vi "TestSequenceSubVI.vi"(0 "GuiRef":T1, 11 "errorin":errorcluster) -> (15 "errorout":errorcluster)   [LabVIEW 2013]
uses:
  Ctl/Paractl.ctl
  GlobValue.vi
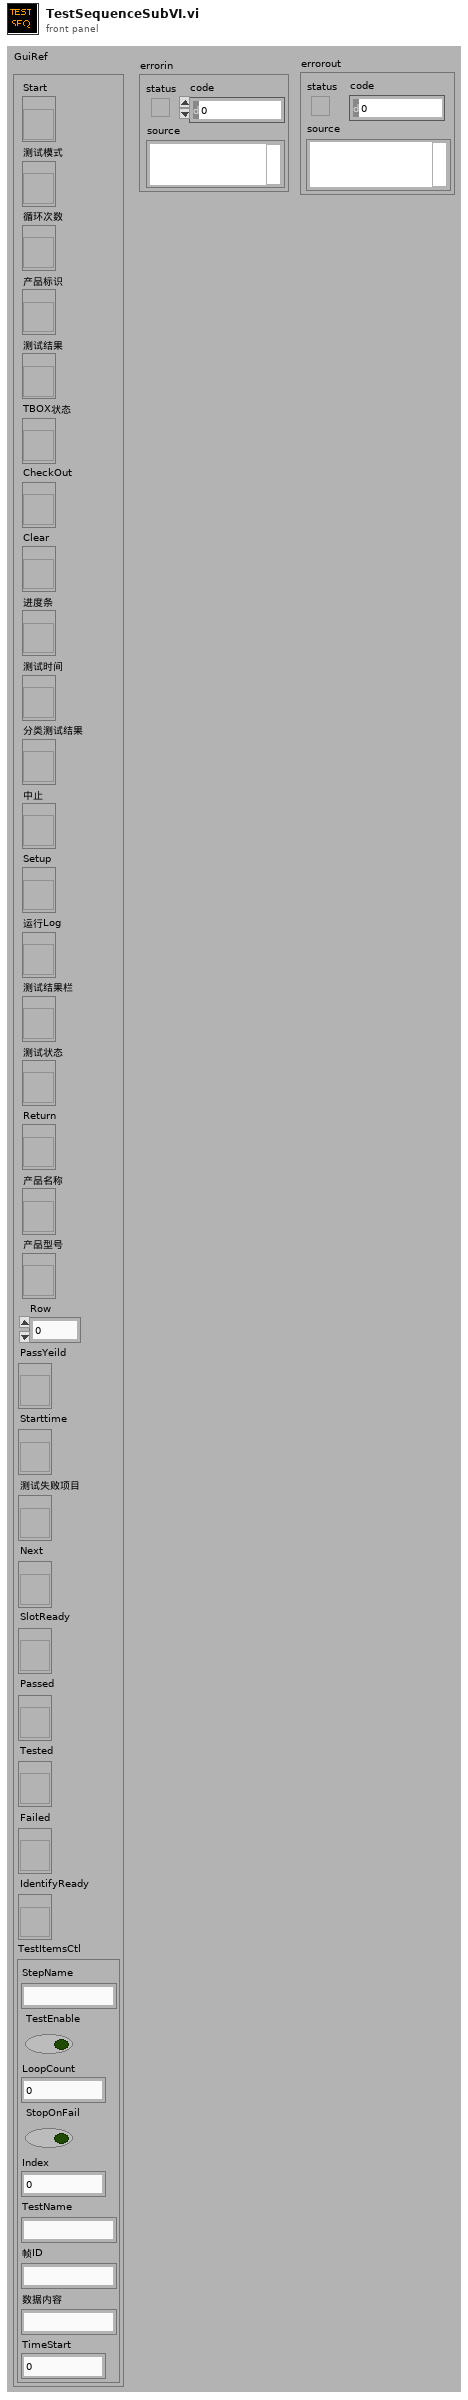
[diagram p1: front panel]
types:
  T1 = typedef "控件.ctl" = cluster{"Start":refnum<vi>, "测试模式":refnum<vi>, "循环次数":refnum<vi>, "产品标识":refnum<vi>, "测试结果":refnum<vi>, "TBOX状态":refnum<vi>, "CheckOut":refnum<vi>, "Clear":refnum<vi>, "进度条":refnum<vi>, "测试时间":refnum<vi>, "分类测试结果":refnum<vi>, "中止":refnum<vi>, "Setup":refnum<vi>, "运行Log":refnum<vi>, "测试结果栏":refnum<vi>, "测试状态":refnum<vi>, "Return":refnum<vi>, "产品名称":refnum<vi>, "产品型号":refnum<vi>, "Row":i32, "PassYeild":refnum<vi>, "Starttime":refnum<vi>, "测试失败项目":refnum<vi>, "Next":refnum<vi>, "SlotReady":refnum<vi>, "Passed":refnum<vi>, "Tested":refnum<vi>, "Failed":refnum<vi>, "IdentifyReady":refnum<vi>, "TestItemsCtl":cluster{"StepName":string, "TestEnable":bool, "LoopCount":u32, "StopOnFail":bool, "Index":u32, "TestName":string, "帧ID":string, "数据内容":string, "TimeStart":u32}}
  T2 = typedef "Paractl.ctl" = enum16{"Fw Ver", "HW Ver", "CCID", "WiFiName", "DevID", "SN", "TUID", "CertifID", "PdTime", "Provider", "WiFiPassword", "Imei", "AuthCode", "Reserved1", "Reserved2", "Reserved3"}
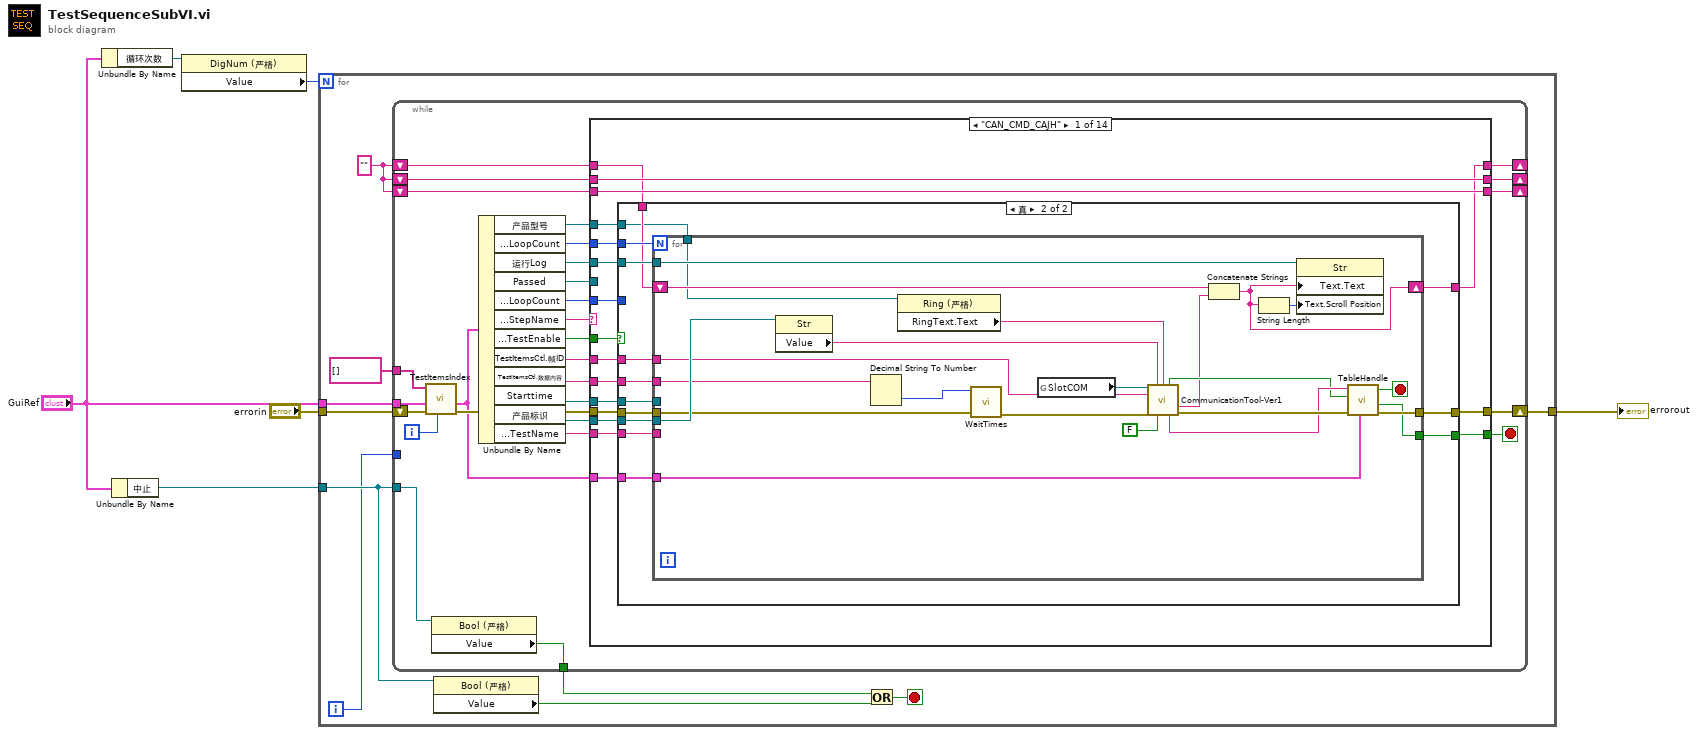
[diagram p0: block diagram]
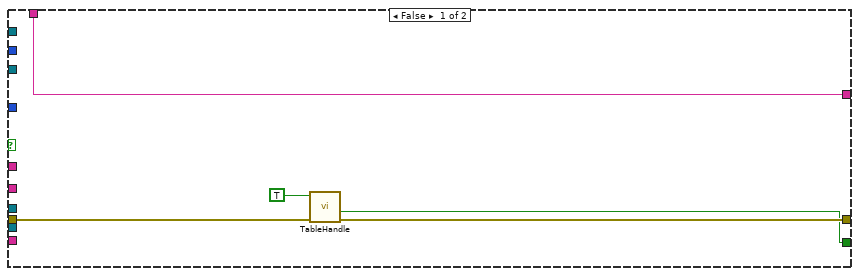
[diagram p2: hidden frame]
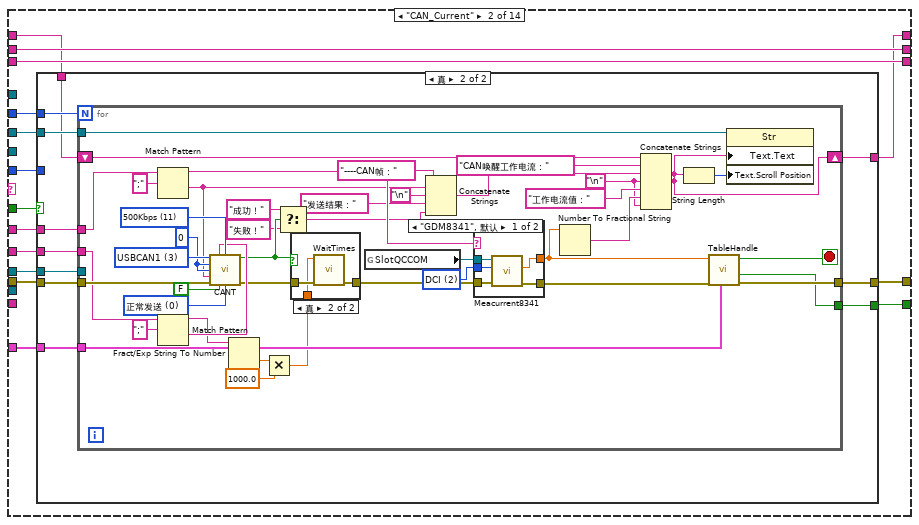
[diagram p3: hidden frame]
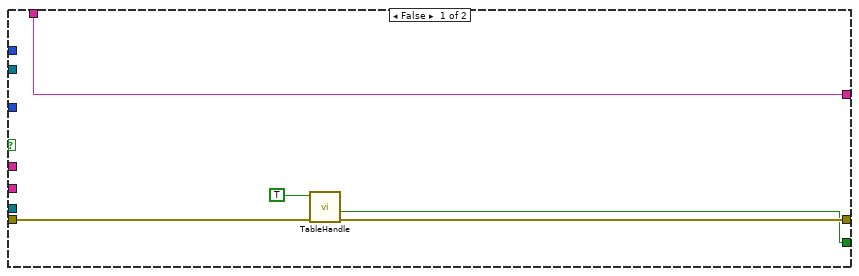
[diagram p4: hidden frame]
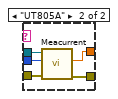
[diagram p6: hidden frame]
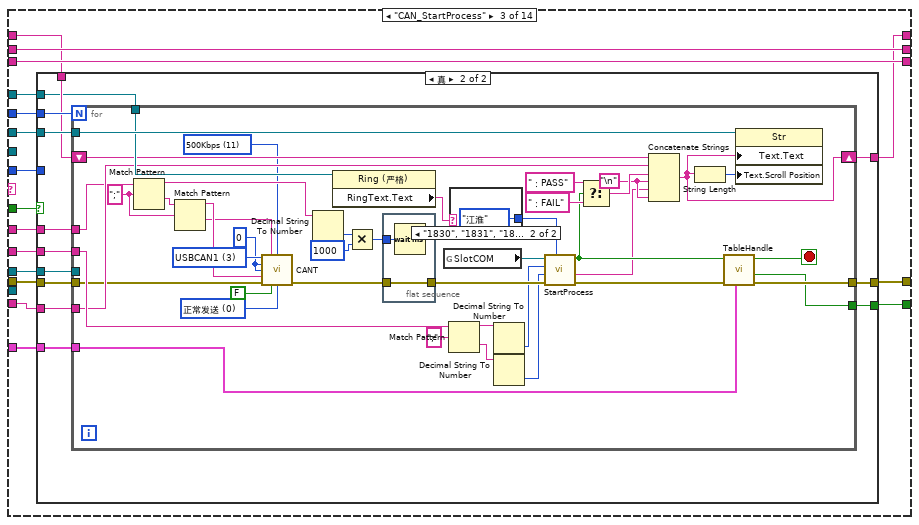
[diagram p7: hidden frame]
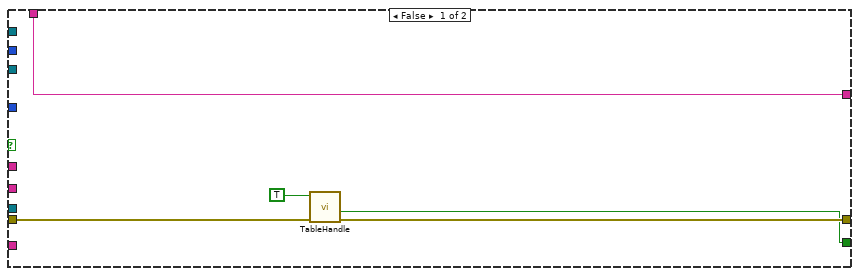
[diagram p8: hidden frame]
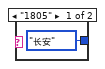
[diagram p9: hidden frame]
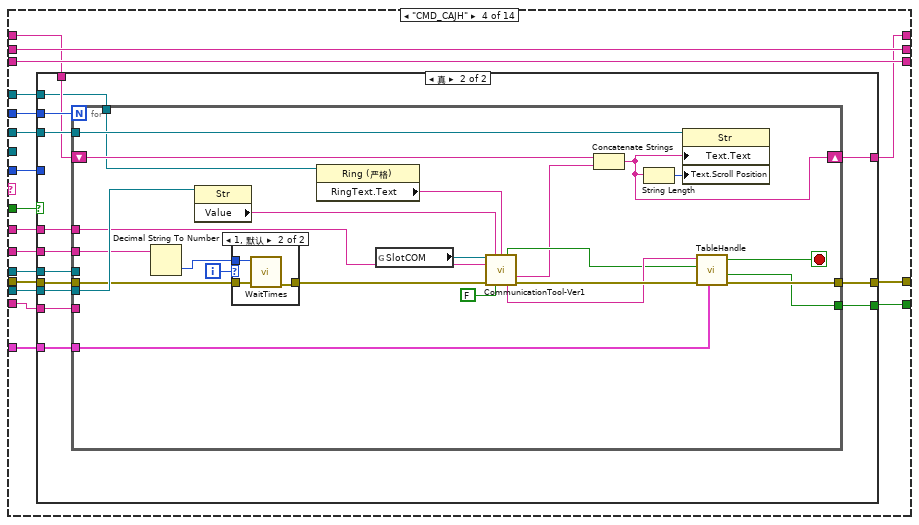
[diagram p10: hidden frame]
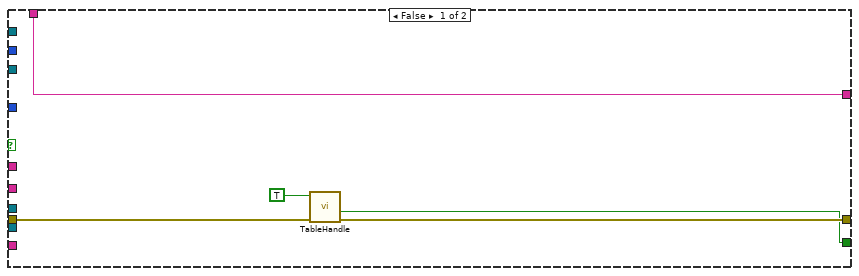
[diagram p11: hidden frame]
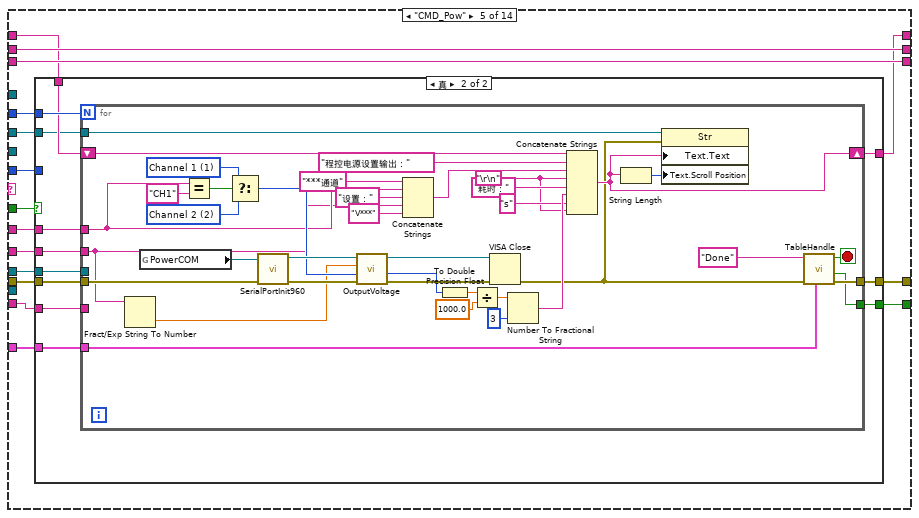
[diagram p13: hidden frame]
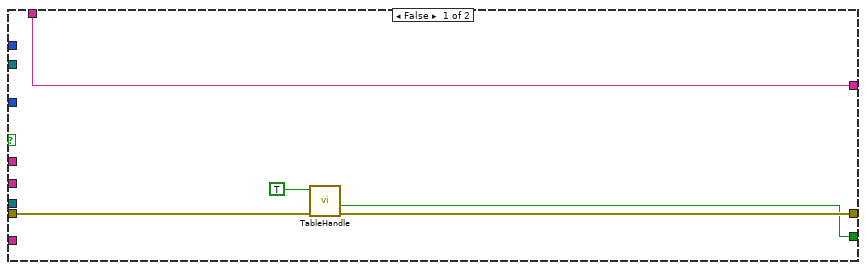
[diagram p14: hidden frame]
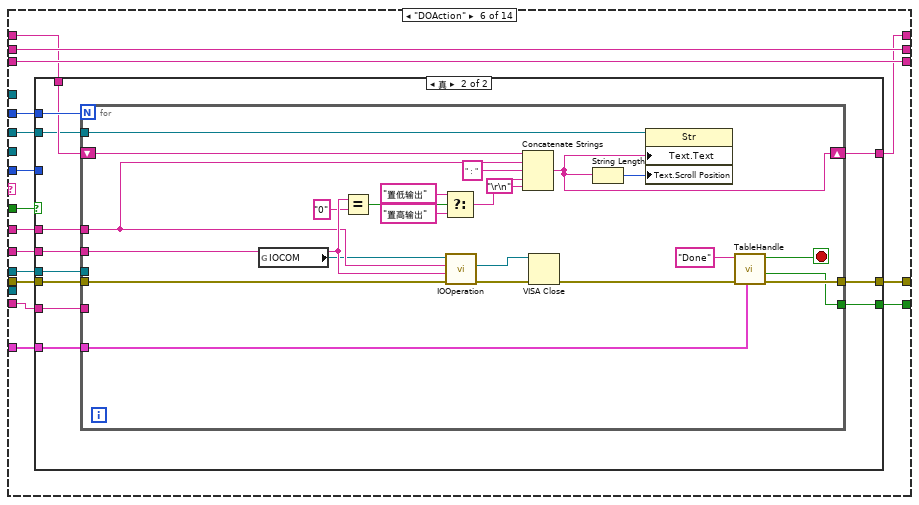
[diagram p15: hidden frame]
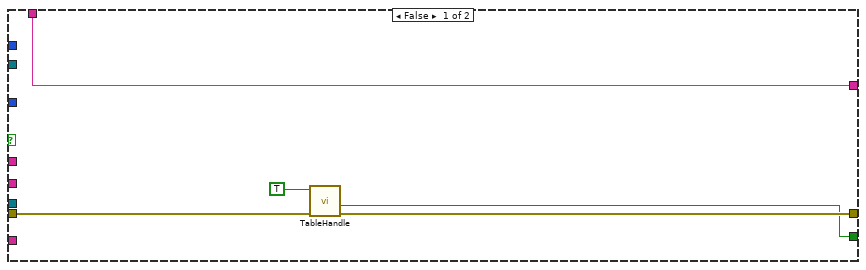
[diagram p16: hidden frame]
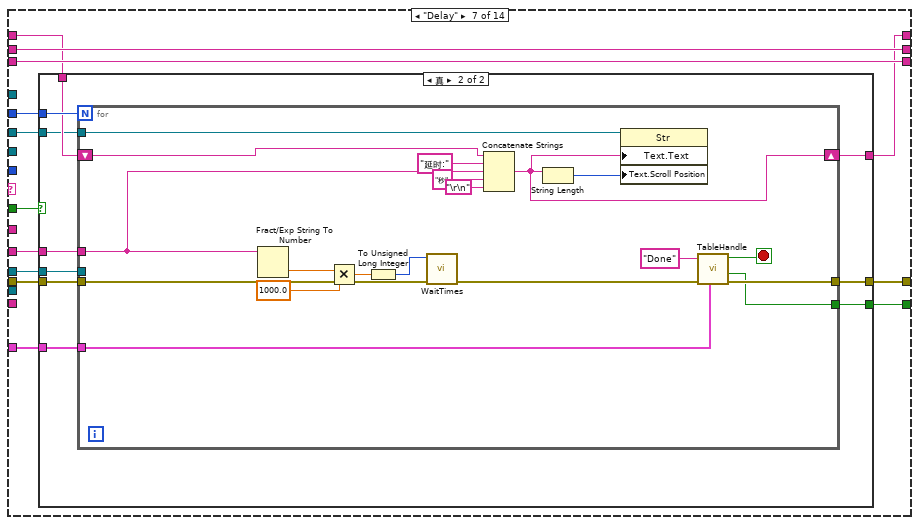
[diagram p17: hidden frame]
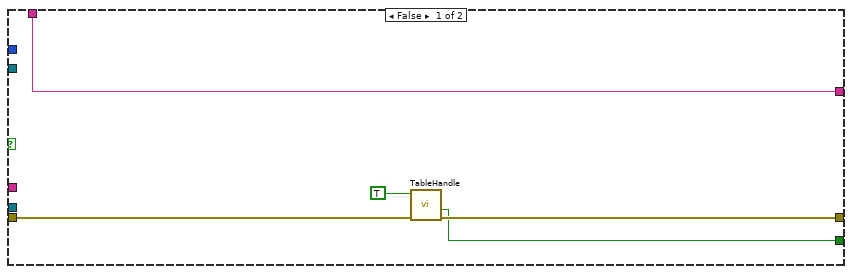
[diagram p18: hidden frame]
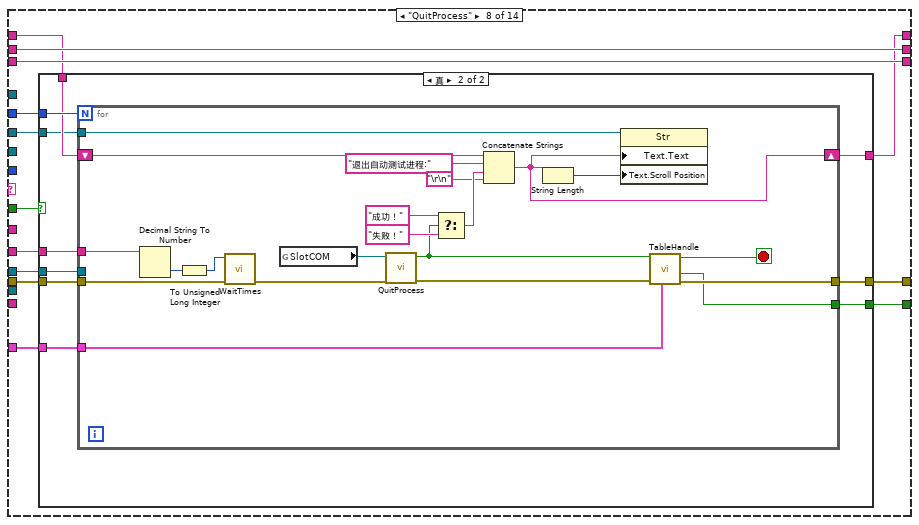
[diagram p19: hidden frame]
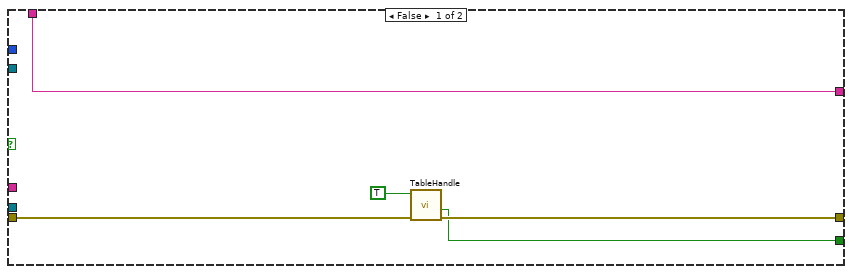
[diagram p20: hidden frame]
diagram:
  n1 = Unbundle By Name("GuiRef") -> ("循环次数"=w4:refnum<vi>)
  n2 = Unbundle By Name("GuiRef") -> ("中止"=w1:refnum<vi>)
  n3 = property class="DigNum (严格)"(reference=w4) -> ("Value"=w3:u32)  [unwired: 1 in, 2 out]
  n4 = for {
    N: w3 -> [_]
    tunnel: [w16] -> w6
    tunnel: "errorin" -> [w15]
    tunnel: "GuiRef" -> [w14]
    tunnel: w1 -> [w11]
    i -> [w7]
    stop <- w8 stop-if-true
    w12 = "" ("CMD")
    n5 = while {
      shift-right: [w40] -> w16
      shift-left: w15 -> [w44]
      tunnel: w14 -> [w19]
      shift-right: [w31] -> _
      shift-left: w12 -> [w30]
      tunnel: string[] [] ("Fail项目") -> [w29]
      shift-right: [w27] -> _
      shift-left: w12 -> [w26]
      shift-right: [w24] -> _
      shift-left: w12 -> [w25]
      tunnel: w11 -> [w18]
      tunnel: [w17] -> w10
      tunnel: w7 -> [_]
      i -> [w28]
      stop <- w39 stop-if-true
      n6 = call "TestItemsIndex.vi"("TestItemIndexIn"=w28, "ErrorIn"=w44, "GuiRef"=w19, "Fail项目"=w29) -> ("ErrorOut"=w43:errorcluster, "GuiRefOut"=w38:T1)  [unwired: 6 in]
      n7 = property class="Bool (严格)"(reference=w18) -> ("Value"=w17:bool)  [unwired: 1 in, 2 out]
      n8 = Unbundle By Name(w38) -> ("产品型号"=w21:refnum<vi>, "TestItemsCtl.LoopCount"=w23:u32, "运行Log"=w32:refnum<vi>, "Passed"=w33:refnum<vi>, "TestItemsCtl.LoopCount"=w34:u32, "TestItemsCtl.StepName"=w42:string, "TestItemsCtl.TestEnable"=w41:bool, "TestItemsCtl.帧ID"=w35:string, "TestItemsCtl.数据内容"=w36:string, "Starttime"=w37:refnum<vi>, "产品标识"=w22:refnum<vi>, "TestItemsCtl.TestName"=w20:string)
      n9 = case shown="\"CAN_CMD_CAJH\"" w42 {
        selector: w42 -> [_ _ _ _ _ _ _ _ _ _ _ _ _ w788]
        tunnel: [w53 w110 w200 w283 w353 w424 w477 w524 w570 w643 w700 w713 w780 w790] -> w40
        tunnel: w43 -> [w57 w114 w204 w287 w354 w425 w478 w525 w574 w647 w700 w714 w780 _]
        tunnel: w38 -> [w56 w113 w203 w286 w355 w426 w479 w526 w573 w646 _ w715 _ _]
        tunnel: w41 -> [w52 w109 w199 w282 w352 w423 w476 w523 w569 w642 _ w712 _ _]
        tunnel: [w54 w111 w201 w284 w351 w422 w475 w522 w571 w644 TRUE ("StopOnFail?") w711 FALSE ("StopOnFail?") TRUE ("StopOnFail?")] -> w39
        tunnel: w37 -> [w55 w112 w202 w285 w350 w421 w474 w521 w572 w645 _ w710 _ _]
        tunnel: w36 -> [w58 w115 w205 w288 w348 w419 w473 w520 w575 w648 _ w708 _ _]
        tunnel: w35 -> [w59 w116 w206 w289 w349 w420 _ _ w576 w649 _ w709 _ _]
        tunnel: w34 -> [w60 w117 w207 w290 w347 w418 _ _ w577 w650 _ _ _ _]
        tunnel: w33 -> [_ _ _ _ _ _ _ _ _ _ _ _ _ _]
        tunnel: w32 -> [w51 w108 w198 w281 w342 w413 w468 w515 w568 w641 _ w704 _ _]
        tunnel: [w48 w105 w195 w278 w340 w411 w467 w514 w565 w638 w698 w703 w778 w785] -> w31
        tunnel: w30 -> [w49 w106 w196 w279 w343 w414 w469 w516 w566 w639 w698 w705 w778 w785]
        tunnel: [w62 w119 w209 w292 w346 w417 w472 w519 w579 w652 w697 w707 w777 w782] -> w27
        tunnel: w26 -> [w62 w119 w209 w292 w346 w417 w472 w519 w579 w652 w697 w707 w777 w782]
        tunnel: w25 -> [w61 w118 w208 w291 w345 w416 w471 w518 w578 w651 w696 w706 w776 w781]
        tunnel: [w61 w118 w208 w291 w345 w416 w471 w518 w578 w651 w696 w706 w776 w781] -> w24
        tunnel: w23 -> [w50 w107 w197 w280 w344 w415 w470 w517 w567 w640 _ w701 _ _]
        tunnel: w22 -> [w45 _ _ w275 _ _ _ _ _ _ _ _ _ _]
        tunnel: w21 -> [w47 _ w194 w277 _ _ _ _ w564 _ _ w702 _ _]
        tunnel: w20 -> [w46 _ w193 w276 w341 w412 _ _ w563 _ _ _ _ _]
        frame "CAN_CMD_CAJH" {
          n10 = case shown="真" w52 {
            tunnel: w56 -> [_ w79]
            tunnel: w57 -> [w66 w81]
            tunnel: [w67 w80] -> w53
            tunnel: [w65 w78] -> w54
            tunnel: w55 -> [_ w77]
            tunnel: w59 -> [_ w76]
            tunnel: w58 -> [_ w75]
            tunnel: w60 -> [_ _]
            tunnel: w51 -> [_ w74]
            tunnel: w50 -> [_ w73]
            tunnel: w49 -> [w63 w72]
            tunnel: [w63 w71] -> w48
            tunnel: w47 -> [_ w70]
            tunnel: w46 -> [_ w69]
            tunnel: w45 -> [_ w68]
            frame False {
              n11 = call "TableHandle.vi"("error in"=w66, "DataIn"=TRUE) -> ("error out"=w67:errorcluster, "Stop?"=w65:bool)  [unwired: 4 in, 4 out]
            }
            frame True {
              n12 = for "For循环" {
                N: w73 -> [_]
                tunnel: w81 -> [w86]
                tunnel: [w104] -> w80
                tunnel: w79 -> [w82]
                tunnel: [w102] -> w78
                tunnel: w77 -> [_]
                tunnel: w75 -> [w84]
                tunnel: w76 -> [w92]
                tunnel: w74 -> [w101]
                shift-right: [w98] -> w71
                shift-left: w72 -> [w100]
                tunnel: w70 -> [w96]
                tunnel: w69 -> [_]
                tunnel: w68 -> [w94]
                stop <- w103 stop-if-true
                n13 = property class="Str"(reference=w94) -> ("Value"=w93:string)  [unwired: 1 in, 2 out]
                n14 = Decimal String To Number(string=w84) -> (number=w83:i32)  [unwired: 2 in, 1 out]
                n15 = property class="Ring (严格)"(reference=w96) -> ("RingText.Text"=w95:string)  [unwired: 1 in, 2 out]
                n16 = call "WaitTimes.vi"("error in (no error)"=w86, "WaitTimes"=w83) -> ("error out"=w85:errorcluster)  [unwired: 9 in]
                n17 = global read "GlobValue.vi" "SlotCOM"() -> (w91:refnum<visa-resource-name>)
                n18 = call "CommunicationTool-Ver1.vi"("VISA资源名称"=w91, "SN"=w93, "ModelNumber"=w95, "通信协议名称"=w92, "error in"=w85, "Debug"=FALSE) -> ("字符串数值"=w88:bool, "CMD"=w87:string, "data"=w89:string, "error out"=w97:errorcluster)  [unwired: 4 in, 2 out]
                n19 = Concatenate Strings(w100, w87) -> (w98:string)
                n20 = String Length(string=w98) -> (length=w99:i32)
                n21 = property class="Str"(reference=w101, "Text.Text"=w98, "Text.Scroll Position"=w99) -> ()  [unwired: 1 in, 2 out]
                n22 = call "TableHandle.vi"("All"=w82, "error in"=w97, "字符串数值"=w88, "DataIn"=w89) -> ("error out"=w104:errorcluster, "Stop?"=w102:bool, "StopForLoop"=w103:bool)  [unwired: 3 in, 2 out]
              }
            }
          }
        }
        frame "CAN_Current" {
          n23 = case shown="真" w109 {
            tunnel: w113 -> [_ w133]
            tunnel: w114 -> [w123 w135]
            tunnel: [w124 w134] -> w110
            tunnel: [w122 w132] -> w111
            tunnel: w112 -> [_ w131]
            tunnel: w116 -> [_ w130]
            tunnel: w115 -> [_ w129]
            tunnel: w117 -> [_ _]
            tunnel: w108 -> [_ w128]
            tunnel: w107 -> [_ w127]
            tunnel: w106 -> [w120 w126]
            tunnel: [w120 w125] -> w105
            frame False {
              n24 = call "TableHandle.vi"("error in"=w123, "DataIn"=TRUE) -> ("error out"=w124:errorcluster, "Stop?"=w122:bool)  [unwired: 4 in, 4 out]
            }
            frame True {
              n25 = for "For循环" {
                N: w127 -> [_]
                tunnel: w135 -> [w166]
                tunnel: [w178] -> w134
                tunnel: w133 -> [w154]
                tunnel: [w176] -> w132
                tunnel: w131 -> [_]
                tunnel: w129 -> [w157]
                tunnel: w130 -> [w160]
                tunnel: w128 -> [w172]
                shift-right: [w167] -> w125
                shift-left: w126 -> [w171]
                stop <- w177 stop-if-true
                w136 = "\n"
                w158 = u32 11 items=["5Kbps", "10Kbps", "20Kbps", "40Kbps", "50Kbps", "80Kbps", "100Kbps", "125Kbps", "200Kbps", "250Kbps", "400Kbps", "500Kbps", "666Kbps", "800Kbps", "1000Kbps"] ("Baud")
                w162 = u8 0 items=["正常发送", "单次发送", "自发自收", "单次自发自收"] ("发送类型")
                w164 = u32 0 ("DevIndex")
                w165 = u32 3 items=["PCI5121"=1, "PCI9810"=2, "USBCAN1"=3, "USBCAN2"=4, "PCI9820"=5, "PCI5110"=7, "PC104CAN"=11, "CANETUDP"=12, "PCI9840B"=14, "PC104C2"=15, "PCI9820I"=16, "CANETTCP"=17, "PCIE9221"=24, "PCI5010U"=19, "USBCAN_E_U"=20, "USBCAN_2E_U"=21, "PCI5020U"=22] ("设备类型")
                w174 = u16 2 items=["DCV", "ACV", "DCI", "ACI", "OHM", "RST", "CAP", "FRQ", "AUTO"] ("测试类型")
                n26 = Match Pattern(string=w160, regular expression=";" ("正则表达式")) -> (before substring=w159:string, after substring=w146:string)  [unwired: 1 in, 2 out]
                n27 = Match Pattern(string=w157, regular expression=";" ("正则表达式")) -> (before substring=w151:string, after substring=w155:string)  [unwired: 1 in, 2 out]
                n28 = call "CANT.vi"("设备类型"=w165, "数据输入"=w155, "Baud"=w158, "DevIndex"=w164, "CANInd"=w164, "ID"=w146, "error in"=w166, "滤波"=FALSE, "发送类型"=w162) -> ("Result"=w145:bool, "error out"=w153:errorcluster)  [unwired: 4 in, 1 out]
                n29 = Fract/Exp String To Number(string=w151) -> (number=w150:dbl)  [unwired: 3 in, 1 out]
                n30 = Multiply(x=w150, y=1000.0) -> (x*y=w148:dbl)
                n31 = Select(t="成功！" ("正则表达式"), s=w145, f="失败！" ("正则表达式")) -> (s? t:f=w140:string)
                n32 = case shown="真" w145 {
                  tunnel: w153 -> [w179 w182]
                  tunnel: [w179 w181] -> w152
                  tunnel: w148 -> [_ w180]
                  frame False {
                  }
                  frame True {
                    n33 = call "WaitTimes.vi"("error in (no error)"=w182, "WaitTimes"=w180) -> ("error out"=w181:errorcluster)  [unwired: 9 in]
                  }
                }
                n34 = global read "GlobValue.vi" "SlotQCCOM"() -> (w175:refnum<visa-resource-name>)
                n35 = Concatenate Strings("----CAN帧：" ("字符串"), w146, "\n", "发送结果：" ("字符串"), w140) -> (w139:string)
                n36 = case shown="\"GDM8341\", 默认" w159 {
                  tunnel: w175 -> [w183 w188]
                  tunnel: w174 -> [w187 w192]
                  tunnel: [w186 w191] -> w169
                  tunnel: [w185 w190] -> w173
                  tunnel: w152 -> [w184 w189]
                  frame "GDM8341", Default {
                    n37 = call "Meacurrent8341.vi"("error in"=w184, "测试类型"=w187, "VISA资源名称"=w183) -> ("错误输出"=w185:errorcluster, "数值"=w186:dbl)  [unwired: 6 in, 1 out]
                  }
                  frame "UT805A" {
                    n38 = call "Meacurrent.vi"("error in"=w189, "测试类型"=w192, "VISA"=w188) -> ("error out"=w190:errorcluster, "数值"=w191:dbl)  [unwired: 7 in]
                  }
                }
                n39 = Number To Fractional String(number=w169) -> (F-format string=w137:string)  [unwired: 3 in]
                n40 = Concatenate Strings(w171, "CAN唤醒工作电流：" ("字符串"), w139, w136, "工作电流值：" ("字符串"), w137, w136) -> (w167:string)
                n41 = String Length(string=w167) -> (length=w168:i32)
                n42 = call "TableHandle.vi"("All"=w154, "error in"=w173, "DataIn"=w169) -> ("error out"=w178:errorcluster, "Stop?"=w176:bool, "StopForLoop"=w177:bool)  [unwired: 4 in, 2 out]
                n43 = property class="Str"(reference=w172, "Text.Text"=w167, "Text.Scroll Position"=w168) -> ()  [unwired: 1 in, 2 out]
              }
            }
          }
        }
        frame "CAN_StartProcess" {
          n44 = case shown="真" w199 {
            tunnel: w203 -> [_ w225]
            tunnel: w204 -> [w213 w227]
            tunnel: [w214 w226] -> w200
            tunnel: [w212 w224] -> w201
            tunnel: w202 -> [_ w223]
            tunnel: w206 -> [_ w222]
            tunnel: w205 -> [_ w221]
            tunnel: w207 -> [_ _]
            tunnel: w198 -> [_ w220]
            tunnel: w197 -> [_ w219]
            tunnel: w196 -> [w210 w218]
            tunnel: [w210 w217] -> w195
            tunnel: w194 -> [_ w216]
            tunnel: w193 -> [_ w215]
            frame False {
              n45 = call "TableHandle.vi"("error in"=w213, "DataIn"=TRUE) -> ("error out"=w214:errorcluster, "Stop?"=w212:bool)  [unwired: 4 in, 4 out]
            }
            frame True {
              n46 = for "For循环" {
                N: w219 -> [_]
                tunnel: w227 -> [w239]
                tunnel: [w270] -> w226
                tunnel: w225 -> [w228]
                tunnel: [w268] -> w224
                tunnel: w223 -> [_]
                tunnel: w221 -> [w257]
                tunnel: w222 -> [w243]
                tunnel: w220 -> [w267]
                shift-right: [w245] -> w217
                shift-left: w218 -> [w249]
                tunnel: w216 -> [w263]
                tunnel: w215 -> [w248]
                stop <- w269 stop-if-true
                w232 = u32 11 items=["5Kbps", "10Kbps", "20Kbps", "40Kbps", "50Kbps", "80Kbps", "100Kbps", "125Kbps", "200Kbps", "250Kbps", "400Kbps", "500Kbps", "666Kbps", "800Kbps", "1000Kbps"] ("Baud")
                w237 = u8 0 items=["正常发送", "单次发送", "自发自收", "单次自发自收"] ("发送类型")
                w240 = u32 0 ("DevIndex")
                w241 = u32 3 items=["PCI5121"=1, "PCI9810"=2, "USBCAN1"=3, "USBCAN2"=4, "PCI9820"=5, "PCI5110"=7, "PC104CAN"=11, "CANETUDP"=12, "PCI9840B"=14, "PC104C2"=15, "PCI9820I"=16, "CANETTCP"=17, "PCIE9221"=24, "PCI5010U"=19, "USBCAN_E_U"=20, "USBCAN_2E_U"=21, "PCI5020U"=22] ("设备类型")
                w235 = ";"
                w251 = "\n"
                n47 = Match Pattern(string=w243, regular expression=w235) -> (before substring=w242:string, after substring=w236:string)  [unwired: 1 in, 2 out]
                n48 = Match Pattern(string=w236, regular expression=w235) -> (before substring=w234:string, after substring=w233:string)  [unwired: 1 in, 2 out]
                n49 = call "CANT.vi"("设备类型"=w241, "数据输入"=w233, "Baud"=w232, "DevIndex"=w240, "CANInd"=w240, "ID"=w234, "error in"=w239, "滤波"=FALSE, "发送类型"=w237) -> ("error out"=w244:errorcluster)  [unwired: 4 in, 2 out]
                n50 = Decimal String To Number(string=w242) -> (number=w231:i32)  [unwired: 2 in, 1 out]
                n51 = property class="Ring (严格)"(reference=w263) -> ("RingText.Text"=w264:string)  [unwired: 1 in, 2 out]
                n52 = Multiply(x=w231, y=1000) -> (x*y=w229:i32)
                n53 = flat-sequence {
                  tunnel: [w272] -> w261
                  tunnel: w244 -> [w272]
                  tunnel: w229 -> [w271]
                  frame #0 {
                    n54 = Wait (ms)(milliseconds to wait=w271) -> ()  [unwired: 1 out]
                  }
                }
                n55 = global read "GlobValue.vi" "SlotCOM"() -> (w265:refnum<visa-resource-name>)
                n56 = Match Pattern(string=w257, regular expression=";") -> (before substring=w259:string, after substring=w258:string)  [unwired: 1 in, 2 out]
                n57 = case shown="\"1830\", \"1831\", \"1832\", 默认" w264 {
                  tunnel: [enum16{"长安", "江淮"}."长安" ("型号") enum16{"长安", "江淮"}."江淮" ("型号")] -> w262
                  frame "1805" {
                  }
                  frame "1830", "1831", "1832", Default {
                  }
                }
                n58 = Decimal String To Number(string=w259) -> (number=w256:i32)  [unwired: 2 in, 1 out]
                n59 = Decimal String To Number(string=w258) -> (number=w255:i32)  [unwired: 2 in, 1 out]
                n60 = call "StartProcess.vi"("型号"=w262, "error in"=w261, "延时"=w255, "Cycles"=w256, "COMIn"=w265) -> ("error out"=w266:errorcluster, "连接的字符串"=w247:string, "OK？"=w250:bool)  [unwired: 3 in, 1 out]
                n61 = Select(t="：PASS", s=w250, f="：FAIL") -> (s? t:f=w252:string)
                n62 = Concatenate Strings(w249, w248, w252, w251, w247, w251) -> (w245:string)
                n63 = String Length(string=w245) -> (length=w246:i32)
                n64 = call "TableHandle.vi"("All"=w228, "error in"=w266, "DataIn"=w250) -> ("error out"=w270:errorcluster, "Stop?"=w268:bool, "StopForLoop"=w269:bool)  [unwired: 4 in, 2 out]
                n65 = property class="Str"(reference=w267, "Text.Text"=w245, "Text.Scroll Position"=w246) -> ()  [unwired: 1 in, 2 out]
              }
            }
          }
        }
        frame "CMD_CAJH" {
          n66 = case shown="真" w282 {
            tunnel: w286 -> [_ w309]
            tunnel: w287 -> [w296 w311]
            tunnel: [w297 w310] -> w283
            tunnel: [w295 w308] -> w284
            tunnel: w285 -> [_ w307]
            tunnel: w289 -> [_ w306]
            tunnel: w288 -> [_ w305]
            tunnel: w290 -> [_ _]
            tunnel: w281 -> [_ w304]
            tunnel: w280 -> [_ w303]
            tunnel: w279 -> [w293 w302]
            tunnel: [w293 w301] -> w278
            tunnel: w277 -> [_ w300]
            tunnel: w276 -> [_ w299]
            tunnel: w275 -> [_ w298]
            frame False {
              n67 = call "TableHandle.vi"("error in"=w296, "DataIn"=TRUE) -> ("error out"=w297:errorcluster, "Stop?"=w295:bool)  [unwired: 4 in, 4 out]
            }
            frame True {
              n68 = for "For循环" {
                N: w303 -> [_]
                tunnel: w311 -> [w317]
                tunnel: [w335] -> w310
                tunnel: w309 -> [w312]
                tunnel: [w333] -> w308
                tunnel: w307 -> [_]
                tunnel: w305 -> [w314]
                tunnel: w306 -> [w323]
                tunnel: w304 -> [w332]
                shift-right: [w329] -> w301
                shift-left: w302 -> [w331]
                tunnel: w300 -> [w327]
                tunnel: w299 -> [_]
                tunnel: w298 -> [w325]
                i -> [w315]
                stop <- w334 stop-if-true
                n69 = Decimal String To Number(string=w314) -> (number=w313:i32)  [unwired: 2 in, 1 out]
                n70 = property class="Str"(reference=w325) -> ("Value"=w324:string)  [unwired: 1 in, 2 out]
                n71 = case shown="1, 默认" w315 {
                  tunnel: w317 -> [w336 w339]
                  tunnel: [w336 w338] -> w316
                  tunnel: w313 -> [_ w337]
                  frame 0 {
                  }
                  frame 1, Default {
                    n72 = call "WaitTimes.vi"("error in (no error)"=w339, "WaitTimes"=w337) -> ("error out"=w338:errorcluster)  [unwired: 9 in]
                  }
                }
                n73 = property class="Ring (严格)"(reference=w327) -> ("RingText.Text"=w326:string)  [unwired: 1 in, 2 out]
                n74 = global read "GlobValue.vi" "SlotCOM"() -> (w322:refnum<visa-resource-name>)
                n75 = call "CommunicationTool-Ver1.vi"("VISA资源名称"=w322, "SN"=w324, "ModelNumber"=w326, "通信协议名称"=w323, "error in"=w316, "Debug"=FALSE) -> ("字符串数值"=w319:bool, "CMD"=w318:string, "data"=w320:string, "error out"=w328:errorcluster)  [unwired: 4 in, 2 out]
                n76 = Concatenate Strings(w331, w318) -> (w329:string)
                n77 = String Length(string=w329) -> (length=w330:i32)
                n78 = property class="Str"(reference=w332, "Text.Text"=w329, "Text.Scroll Position"=w330) -> ()  [unwired: 1 in, 2 out]
                n79 = call "TableHandle.vi"("All"=w312, "error in"=w328, "字符串数值"=w319, "DataIn"=w320) -> ("error out"=w335:errorcluster, "Stop?"=w333:bool, "StopForLoop"=w334:bool)  [unwired: 3 in, 2 out]
              }
            }
          }
        }
        frame "CMD_Pow" {
          n80 = case shown="真" w352 {
            tunnel: w355 -> [_ w370]
            tunnel: w354 -> [w359 w372]
            tunnel: [w360 w371] -> w353
            tunnel: [w358 w369] -> w351
            tunnel: w350 -> [_ w368]
            tunnel: w349 -> [_ w367]
            tunnel: w348 -> [_ w366]
            tunnel: w347 -> [_ _]
            tunnel: w344 -> [_ w365]
            tunnel: w343 -> [w356 w364]
            tunnel: w342 -> [_ w363]
            tunnel: w341 -> [_ w362]
            tunnel: [w356 w361] -> w340
            frame False {
              n81 = call "TableHandle.vi"("error in"=w359, "DataIn"=TRUE) -> ("error out"=w360:errorcluster, "Stop?"=w358:bool)  [unwired: 4 in, 4 out]
            }
            frame True {
              n82 = for "For循环" {
                N: w365 -> [_]
                tunnel: w372 -> [w405]
                tunnel: [w410] -> w371
                tunnel: w370 -> [w374]
                tunnel: [w408] -> w369
                tunnel: w368 -> [_]
                tunnel: w366 -> [w386]
                tunnel: w367 -> [w388]
                shift-right: [w401] -> w361
                shift-left: w364 -> [w403]
                tunnel: w363 -> [w404]
                tunnel: w362 -> [_]
                stop <- w409 stop-if-true
                w395 = 2 items=["Channel 1"=1, "Channel 2"=2] ("Channel")
                w396 = 1 items=["Channel 1"=1, "Channel 2"=2] ("Channel")
                w375 = "\r\n"
                n83 = Fract/Exp String To Number(string=w386) -> (number=w392:dbl)  [unwired: 3 in, 1 out]
                n84 = global read "GlobValue.vi" "PowerCOM"() -> (w406:refnum<visa-resource-name>)
                n85 = Equal?(x=w388, y="CH1") -> (x = y?=w397:bool)
                n86 = Select(t=w396, s=w397, f=w395) -> (s? t:f=w394:i32)
                n87 = call "SerialPortInit960.vi"("错误输入"=w405, "COMIn"=w406) -> ("错误输出"=w393:errorcluster, "COMOut"=w400:refnum<visa-resource-name>)  [unwired: 8 in]
                n88 = call "OutputVoltage.vi"("error in"=w393, "Channel"=w394, "Voltage Level"=w392, "VISAin"=w400) -> ("error out"=w399:errorcluster, "time"=w382:u32, "VISAout"=w391:refnum<visa-resource-name>)  [unwired: 5 in]
                n89 = Concatenate Strings("***通道", w388, "设置：", w386, "V***") -> (w384:string)
                n90 = To Double Precision Float(number=w382) -> (double precision float=w381:dbl)
                n91 = Divide(x=w381, y=1000.0) -> (x/y=w379:dbl)
                n92 = VISA Close(VISA resource name=w391, error in (no error)=w399) -> (error out=w373:errorcluster)
                n93 = Number To Fractional String(number=w379, precision (6)=i16 3 ("精度(6)")) -> (F-format string=w377:string)  [unwired: 2 in]
                n94 = Concatenate Strings(w403, "程控电源设置输出：", w384, w375, "耗时：" ("字符串"), w377, "s" ("字符串"), w375) -> (w401:string)
                n95 = String Length(string=w401) -> (length=w402:i32)
                n96 = property class="Str"(reference=w404, error in=w373, "Text.Text"=w401, "Text.Scroll Position"=w402) -> ()  [unwired: 2 out]
                n97 = call "TableHandle.vi"("All"=w374, "error in"=w373, "DataIn"="Done") -> ("error out"=w410:errorcluster, "Stop?"=w408:bool, "StopForLoop"=w409:bool)  [unwired: 4 in, 2 out]
              }
            }
          }
        }
        frame "DOAction" {
          n98 = case shown="真" w423 {
            tunnel: w426 -> [_ w441]
            tunnel: w425 -> [w430 w443]
            tunnel: [w431 w442] -> w424
            tunnel: [w429 w440] -> w422
            tunnel: w421 -> [_ w439]
            tunnel: w420 -> [_ w438]
            tunnel: w419 -> [_ w437]
            tunnel: w418 -> [_ _]
            tunnel: w415 -> [_ w436]
            tunnel: w414 -> [w427 w435]
            tunnel: w413 -> [_ w434]
            tunnel: w412 -> [_ w433]
            tunnel: [w427 w432] -> w411
            frame False {
              n99 = call "TableHandle.vi"("error in"=w430, "DataIn"=TRUE) -> ("error out"=w431:errorcluster, "Stop?"=w429:bool)  [unwired: 4 in, 4 out]
            }
            frame True {
              n100 = for "For循环" {
                N: w436 -> [_]
                tunnel: w443 -> [w445]
                tunnel: [w466] -> w442
                tunnel: w441 -> [w446]
                tunnel: [w464] -> w440
                tunnel: w439 -> [_]
                tunnel: w437 -> [w457]
                tunnel: w438 -> [w453]
                shift-right: [w447] -> w432
                shift-left: w435 -> [w458]
                tunnel: w434 -> [w459]
                tunnel: w433 -> [_]
                stop <- w465 stop-if-true
                n101 = global read "GlobValue.vi" "IOCOM"() -> (w444:refnum<visa-resource-name>)
                n102 = Equal?(x=w457, y="0") -> (x = y?=w455:bool)
                n103 = Select(t="置低输出" ("y"), s=w455, f="置高输出" ("y")) -> (s? t:f=w450:string)
                n104 = call "IOOperation.vi"("error in"=w445, "Value"=w457, "Channel"=w453, "Com"=w444) -> ("error out"=w462:errorcluster, "ComOut"=w461:refnum<visa-resource-name>)  [unwired: 5 in, 1 out]
                n105 = Concatenate Strings(w458, w453, "：" ("字符串"), w450, "\r\n") -> (w447:string)
                n106 = VISA Close(VISA resource name=w461, error in (no error)=w462) -> (error out=w460:errorcluster)
                n107 = String Length(string=w447) -> (length=w448:i32)
                n108 = property class="Str"(reference=w459, "Text.Text"=w447, "Text.Scroll Position"=w448) -> ()  [unwired: 1 in, 2 out]
                n109 = call "TableHandle.vi"("All"=w446, "error in"=w460, "DataIn"="Done") -> ("error out"=w466:errorcluster, "Stop?"=w464:bool, "StopForLoop"=w465:bool)  [unwired: 4 in, 2 out]
              }
            }
          }
        }
        frame "Delay" {
          n110 = case shown="真" w476 {
            tunnel: w479 -> [_ w492]
            tunnel: w478 -> [w483 w494]
            tunnel: [w484 w493] -> w477
            tunnel: [w482 w491] -> w475
            tunnel: w474 -> [_ w490]
            tunnel: w473 -> [_ w489]
            tunnel: w470 -> [_ w488]
            tunnel: w469 -> [w480 w487]
            tunnel: w468 -> [_ w486]
            tunnel: [w480 w485] -> w467
            frame False {
              n111 = call "TableHandle.vi"("error in"=w483, "DataIn"=TRUE) -> ("error out"=w484:errorcluster, "Stop?"=w482:bool)  [unwired: 4 in, 4 out]
            }
            frame True {
              n112 = for "For循环" {
                N: w488 -> [_]
                tunnel: w494 -> [w510]
                tunnel: [w513] -> w493
                tunnel: w492 -> [w496]
                tunnel: [w511] -> w491
                tunnel: w490 -> [_]
                tunnel: w489 -> [w502]
                shift-right: [w498] -> w485
                shift-left: w487 -> [w495]
                tunnel: w486 -> [w504]
                stop <- w512 stop-if-true
                n113 = Fract/Exp String To Number(string=w502) -> (number=w506:dbl)  [unwired: 3 in, 1 out]
                n114 = Multiply(x=w506, y=1000.0) -> (x*y=w505:dbl)
                n115 = To Unsigned Long Integer(number=w505) -> (unsigned 32bit integer=w497:u32)
                n116 = call "WaitTimes.vi"("error in (no error)"=w510, "WaitTimes"=w497) -> ("error out"=w509:errorcluster)  [unwired: 9 in]
                n117 = Concatenate Strings(w495, "延时:" ("字符串"), w502, "秒" ("字符串"), "\r\n") -> (w498:string)
                n118 = String Length(string=w498) -> (length=w499:i32)
                n119 = property class="Str"(reference=w504, "Text.Text"=w498, "Text.Scroll Position"=w499) -> ()  [unwired: 1 in, 2 out]
                n120 = call "TableHandle.vi"("All"=w496, "error in"=w509, "DataIn"="Done") -> ("error out"=w513:errorcluster, "Stop?"=w511:bool, "StopForLoop"=w512:bool)  [unwired: 6 in]
              }
            }
          }
        }
        frame "QuitProcess" {
          n121 = case shown="真" w523 {
            tunnel: w526 -> [_ w539]
            tunnel: w525 -> [w530 w541]
            tunnel: [w531 w540] -> w524
            tunnel: [w529 w538] -> w522
            tunnel: w521 -> [_ w537]
            tunnel: w520 -> [_ w536]
            tunnel: w517 -> [_ w535]
            tunnel: w516 -> [w527 w534]
            tunnel: w515 -> [_ w533]
            tunnel: [w527 w532] -> w514
            frame False {
              n122 = call "TableHandle.vi"("error in"=w530, "DataIn"=TRUE) -> ("error out"=w531:errorcluster, "Stop?"=w529:bool)  [unwired: 4 in, 4 out]
            }
            frame True {
              n123 = for "For循环" {
                N: w535 -> [_]
                tunnel: w541 -> [w559]
                tunnel: [w562] -> w540
                tunnel: w539 -> [w553]
                tunnel: [w560] -> w538
                tunnel: w537 -> [_]
                tunnel: w536 -> [w551]
                shift-right: [w555] -> w532
                shift-left: w534 -> [w552]
                tunnel: w533 -> [w558]
                stop <- w561 stop-if-true
                n124 = Decimal String To Number(string=w551) -> (number=w550:i32)  [unwired: 2 in, 1 out]
                n125 = To Unsigned Long Integer(number=w550) -> (unsigned 32bit integer=w554:u32)
                n126 = call "WaitTimes.vi"("error in (no error)"=w559, "WaitTimes"=w554) -> ("error out"=w548:errorcluster)  [unwired: 9 in]
                n127 = global read "GlobValue.vi" "SlotCOM"() -> (w549:refnum<visa-resource-name>)
                n128 = call "QuitProcess.vi"("error in"=w548, "ComIn"=w549) -> ("error out"=w547:errorcluster, "OK？"=w544:bool)  [unwired: 7 in, 1 out]
                n129 = Select(t="成功！", s=w544, f="失败！") -> (s? t:f=w543:string)
                n130 = Concatenate Strings(w552, "退出自动测试进程:" ("字符串"), w543, "\r\n") -> (w555:string)
                n131 = String Length(string=w555) -> (length=w556:i32)
                n132 = property class="Str"(reference=w558, "Text.Text"=w555, "Text.Scroll Position"=w556) -> ()  [unwired: 1 in, 2 out]
                n133 = call "TableHandle.vi"("All"=w553, "error in"=w547, "DataIn"=w544) -> ("error out"=w562:errorcluster, "Stop?"=w560:bool, "StopForLoop"=w561:bool)  [unwired: 6 in]
              }
            }
          }
        }
        frame "StartProcess" {
          n134 = case shown="真" w569 {
            tunnel: w573 -> [_ w595]
            tunnel: w574 -> [w583 w597]
            tunnel: [w584 w596] -> w570
            tunnel: [w582 w594] -> w571
            tunnel: w572 -> [_ w593]
            tunnel: w576 -> [_ w592]
            tunnel: w575 -> [_ w591]
            tunnel: w577 -> [_ _]
            tunnel: w568 -> [_ w590]
            tunnel: w567 -> [_ w589]
            tunnel: w566 -> [w580 w588]
            tunnel: [w580 w587] -> w565
            tunnel: w564 -> [_ w586]
            tunnel: w563 -> [_ w585]
            frame False {
              n135 = call "TableHandle.vi"("error in"=w583, "DataIn"=TRUE) -> ("error out"=w584:errorcluster, "Stop?"=w582:bool)  [unwired: 4 in, 4 out]
            }
            frame True {
              n136 = for "For循环" {
                N: w589 -> [_]
                tunnel: w597 -> [w619]
                tunnel: [w629] -> w596
                tunnel: w595 -> [w598]
                tunnel: [w627] -> w594
                tunnel: w593 -> [_]
                tunnel: w591 -> [w611]
                tunnel: w592 -> [w618]
                tunnel: w590 -> [w626]
                shift-right: [w599] -> w587
                shift-left: w588 -> [w603]
                tunnel: w586 -> [w622]
                tunnel: w585 -> [w602]
                i -> [w615]
                stop <- w628 stop-if-true
                w605 = "\n"
                n137 = Decimal String To Number(string=w618) -> (number=w617:i32)  [unwired: 2 in, 1 out]
                n138 = Greater Than 0?(x=w615) -> (x > 0?=w616:bool)
                n139 = case shown="真" w616 {
                  tunnel: [w630 w633] -> w620
                  tunnel: w619 -> [w630 w632]
                  tunnel: w617 -> [_ w631]
                  frame False {
                  }
                  frame True {
                    n140 = flat-sequence {
                      tunnel: [w635] -> w633
                      tunnel: w632 -> [w635]
                      tunnel: w631 -> [w634]
                      frame #0 {
                        n141 = Wait (ms)(milliseconds to wait=w634) -> ()  [unwired: 1 out]
                      }
                    }
                  }
                }
                n142 = property class="Ring (严格)"(reference=w622) -> ("RingText.Text"=w623:string)  [unwired: 1 in, 2 out]
                n143 = global read "GlobValue.vi" "SlotCOM"() -> (w624:refnum<visa-resource-name>)
                n144 = Match Pattern(string=w611, regular expression=";") -> (before substring=w613:string, after substring=w612:string)  [unwired: 1 in, 2 out]
                n145 = Decimal String To Number(string=w612) -> (number=w609:i32)  [unwired: 2 in, 1 out]
                n146 = Decimal String To Number(string=w613) -> (number=w610:i32)  [unwired: 2 in, 1 out]
                n147 = case shown="\"1830\", \"1831\", \"1832\", 默认" w623 {
                  tunnel: [enum16{"长安", "江淮"}."长安" ("型号") enum16{"长安", "江淮"}."江淮" ("型号")] -> w621
                  frame "1805" {
                  }
                  frame "1830", "1831", "1832", Default {
                  }
                }
                n148 = call "StartProcess.vi"("型号"=w621, "error in"=w620, "延时"=w609, "Cycles"=w610, "COMIn"=w624) -> ("error out"=w625:errorcluster, "连接的字符串"=w601:string, "OK？"=w604:bool)  [unwired: 3 in, 1 out]
                n149 = Select(t="：PASS", s=w604, f="：FAIL") -> (s? t:f=w606:string)
                n150 = Concatenate Strings(w603, w602, w606, w605, w601, w605) -> (w599:string)
                n151 = String Length(string=w599) -> (length=w600:i32)
                n152 = call "TableHandle.vi"("All"=w598, "error in"=w625, "DataIn"=w604) -> ("error out"=w629:errorcluster, "Stop?"=w627:bool, "StopForLoop"=w628:bool)  [unwired: 4 in, 2 out]
                n153 = property class="Str"(reference=w626, "Text.Text"=w599, "Text.Scroll Position"=w600) -> ()  [unwired: 1 in, 2 out]
              }
            }
          }
        }
        frame "Static Current" {
          n154 = case shown="真" w642 {
            tunnel: w646 -> [_ w666]
            tunnel: w647 -> [w656 w668]
            tunnel: [w657 w667] -> w643
            tunnel: [w655 w665] -> w644
            tunnel: w645 -> [_ w664]
            tunnel: w649 -> [_ w663]
            tunnel: w648 -> [_ w662]
            tunnel: w650 -> [_ _]
            tunnel: w641 -> [_ w661]
            tunnel: w640 -> [_ w660]
            tunnel: w639 -> [w653 w659]
            tunnel: [w653 w658] -> w638
            frame False {
              n155 = call "TableHandle.vi"("error in"=w656, "DataIn"=TRUE) -> ("error out"=w657:errorcluster, "Stop?"=w655:bool)  [unwired: 4 in, 4 out]
            }
            frame True {
              n156 = for "For循环" {
                N: w660 -> [_]
                tunnel: w668 -> [w678]
                tunnel: [w685] -> w667
                tunnel: w666 -> [w669]
                tunnel: [w683] -> w665
                tunnel: w664 -> [_]
                tunnel: w662 -> [_]
                tunnel: w663 -> [w680]
                tunnel: w661 -> [w677]
                shift-right: [w670] -> w658
                shift-left: w659 -> [w676]
                stop <- w684 stop-if-true
                w681 = u16 2 items=["DCV", "ACV", "DCI", "ACI", "OHM", "RST", "CAP", "FRQ", "AUTO"] ("测试类型")
                n157 = global read "GlobValue.vi" "SlotQCCOM"() -> (w682:refnum<visa-resource-name>)
                n158 = case shown="\"GDM8341\", 默认" w680 {
                  tunnel: w682 -> [w686 w691]
                  tunnel: w681 -> [w690 w695]
                  tunnel: [w689 w694] -> w674
                  tunnel: [w688 w693] -> w679
                  tunnel: w678 -> [w687 w692]
                  frame "GDM8341", Default {
                    n159 = call "Meacurrent8341.vi"("error in"=w687, "测试类型"=w690, "VISA资源名称"=w686) -> ("错误输出"=w688:errorcluster, "数值"=w689:dbl)  [unwired: 6 in, 1 out]
                  }
                  frame "UT805A" {
                    n160 = call "Meacurrent.vi"("error in"=w692, "测试类型"=w695, "VISA"=w691) -> ("error out"=w693:errorcluster, "数值"=w694:dbl)  [unwired: 7 in]
                  }
                }
                n161 = Number To Fractional String(number=w674) -> (F-format string=w673:string)  [unwired: 3 in]
                n162 = Concatenate Strings(w676, "静态电流值：" ("字符串"), w673, "\r\n") -> (w670:string)
                n163 = String Length(string=w670) -> (length=w672:i32)
                n164 = property class="Str"(reference=w677, "Text.Text"=w670, "Text.Scroll Position"=w672) -> ()  [unwired: 1 in, 2 out]
                n165 = call "TableHandle.vi"("All"=w669, "error in"=w679, "DataIn"=w674) -> ("error out"=w685:errorcluster, "Stop?"=w683:bool, "StopForLoop"=w684:bool)  [unwired: 4 in, 2 out]
              }
            }
          }
        }
        frame "StopTest" {
          # "此步骤不能删除"
        }
        frame "WIFI_DOS" {
          n166 = case shown="真" w712 {
            tunnel: w715 -> [_ w730]
            tunnel: w714 -> [w719 w732]
            tunnel: [w720 w731] -> w713
            tunnel: [w718 w729] -> w711
            tunnel: w710 -> [_ w728]
            tunnel: w709 -> [_ w727]
            tunnel: w708 -> [_ w726]
            tunnel: w705 -> [w716 w725]
            tunnel: w704 -> [_ w724]
            tunnel: [w716 w723] -> w703
            tunnel: w702 -> [_ w722]
            tunnel: w701 -> [_ w721]
            frame False {
              n167 = call "TableHandle.vi"("error in"=w719, "DataIn"=TRUE) -> ("error out"=w720:errorcluster, "Stop?"=w718:bool)  [unwired: 4 in, 4 out]
            }
            frame True {
              n168 = for "For循环" {
                N: w721 -> [_]
                tunnel: w732 -> [w769]
                tunnel: [w772] -> w731
                tunnel: w730 -> [w733]
                tunnel: [w770] -> w729
                tunnel: w728 -> [_]
                tunnel: w726 -> [w740]
                tunnel: w727 -> [w745]
                shift-right: [w753] -> w723
                shift-left: w725 -> [w756]
                tunnel: w724 -> [w755]
                tunnel: w722 -> [w735]
                i -> [w752]
                stop <- w771 stop-if-true
                w749 = "\n"
                n169 = property class="Ring (严格)"(reference=w735) -> ("RingText.Text"=w734:string)  [unwired: 1 in, 2 out]
                n170 = Match Pattern(string=w740, regular expression=";") -> (before substring=w739:string, after substring=w738:string)  [unwired: 1 in, 2 out]
                n171 = Match Pattern(string=w745, regular expression=";") -> (before substring=w743:string, after substring=w742:string)  [unwired: 1 in, 2 out]
                n172 = Fract/Exp String To Number(string=w739) -> (number=w767:dbl)  [unwired: 3 in, 1 out]
                n173 = Multiply(x=w767, y=1000.0) -> (x*y=w766:dbl)
                n174 = Decimal String To Number(string=w738) -> (number=w737:i32)  [unwired: 2 in, 1 out]
                n175 = To Unsigned Long Integer(number=w766) -> (unsigned 32bit integer=w760:u32)
                n176 = case shown="1, 默认" w752 {
                  tunnel: w769 -> [w773 w775]
                  tunnel: w760 -> [_ _]
                  tunnel: [w773 w774] -> w759
                  frame 0 {
                  }
                  frame 1, Default {
                    n177 = call "WaitTimes.vi"("error in (no error)"=w775) -> ("error out"=w774:errorcluster)  [unwired: 10 in]
                  }
                }
                n178 = call "ccidinfo-r.vi"("Data Type"=Paractl."WiFiName") -> ("Data"=w747:string)
                n179 = call "ccidinfo-r.vi"("Data Type"=Paractl."WiFiPassword") -> ("Data"=w746:string)
                n180 = call "WiFi.vi"("New WIFI Name"=w747, "Delay Time (s)"=0.5, "配置连接次数"=w737, "Delay"=w743, "password"=w746, "error in"=w759, "ping次数"=w742, "ModelNumber"=w734) -> ("Acess"=w758:bool, "TotalOut"=w748:string, "error out"=w757:errorcluster)  [unwired: 5 in]
                n181 = Concatenate Strings(w756, "WIFI名:", w747, w749, "WIFI密码:", w746, w749, w748) -> (w753:string)
                n182 = String Length(string=w753) -> (length=w754:i32)
                n183 = Select(t="PASS", s=w758, f="FAIL") -> (s? t:f=w765:string)
                n184 = property class="Str"(reference=w755, "Value"=w753, "Text.Scroll Position"=w754) -> ()  [unwired: 1 in, 2 out]
                n185 = call "TableHandle.vi"("All"=w733, "error in"=w757, "DataIn"=w765) -> ("error out"=w772:errorcluster, "Stop?"=w770:bool, "StopForLoop"=w771:bool)  [unwired: 4 in, 2 out]
              }
            }
          }
        }
        frame "Wait" {
        }
        frame "空", Default {
          # "此步骤不能删除"
          n186 = Concatenate Strings("测试队列 " ("字符串"), "Cann't find the \"" ("source"), w788, "\" item." ("字符串")) -> (w787:string)
          n187 = Bundle By Name(cluster=errorcluster {"status"=TRUE, "code"=5000, "source"=""} ("error in 1 (no error)"), "source"=w787) -> (w790:errorcluster)
        }
      }
    }
    n188 = property class="Bool (严格)"(reference=w11) -> ("Value"=w9:bool)  [unwired: 1 in, 2 out]
    n189 = Or(x=w10, y=w9) -> (x .or. y?=w8:bool)
  }
  "errorout" <- w6
